vi "PH_Stepmotor_BaseClass.PC Relative Move.vi"(0 "i ref in":refnum<vi>, 1 "axis":i32=-1, 3 "Direction":T1, 4 "Multiple":i32=1, 5 "error in (no error)":errorcluster) -> (14 "i ref out":refnum<vi>, 19 "error out":errorcluster)   [LabVIEW 2014, in "PH_Stepmotor_BaseClass.lvlib"]
doc: "This VI calculates the target position and stores it own attributes."
uses:
  PH_Stepmotor_BaseClass.lvlib
  PH_Stepmotor_BaseClass.Axis Direction.ctl
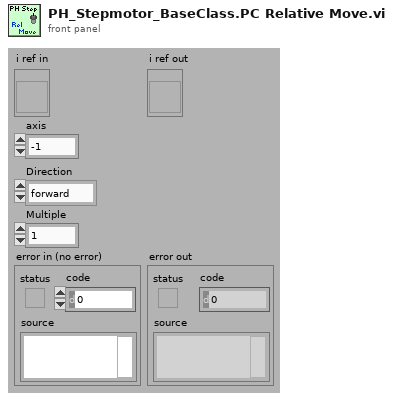
[diagram p1: front panel]
types:
  T1 = typedef "PH_Stepmotor_BaseClass.lvlib/PH_Stepmotor_BaseClass.Axis Direction.ctl" = enum16{"forward", "backward"}
  T2 = typedef "PH_Stepmotor_BaseClass.lvlib/PH_Stepmotor_BaseClass.Axis Attributes.ctl" = cluster{"Settings":T3, "Endswitch?":bool, "DIM Service IDs":T5, "Activity":T6, "Configured?":bool, "Position":cluster{"Current":i32, "Target":i32}, "Position to set":cluster{"New?":bool, "Wanted":i32}, "Stop?":bool, "Reset?":bool, "Move?":bool, "Nothing connected?":bool}
  T3 = typedef "PH_Stepmotor_BaseClass.lvlib/PH_Stepmotor_BaseClass.Axis Settings.ctl" = cluster{"Sign change":bool, "Width":dbl, "Calibration":dbl, "Unit":string, "Motor Type":T4, "Unit Width":string, "Unit CF":string}
  T4 = typedef "PH_Stepmotor_BaseClass.lvlib/PH_Stepmotor_BaseClass.Motor Type.ctl" = enum16{"Unspecific", "OWIS 49.120.2633", "OWIS 49.060.1033", "OWIS 43.040.2558", "Diamond Motion 2200 series", "OWIS 49.120.266B.MV6", "Calorimeter", "Linear Stage 1", "MICOS VT-80", "MICOS VT-80 S", "Standa Rotstage nt0.95A", "PUF RA 320.200", "PUF RA 800.200", "PUF RA 800.400", "PUF RA 400.50", "1324.nn.800.50", "1324.n9c.800.50", "1324.nn.320.200", "1324.nn.400.200", "1324.nn.800.200", "1324.nn.400.50", "1324.8c9c.800.50", "1324.8c9c.400.200"}
  T5 = typedef "PH_Stepmotor_BaseClass.lvlib/PH_Stepmotor_BaseClass.Axis DIM Service IDs.ctl" = cluster{"Settings":i32, "Information":i32}
  T6 = typedef "PH_Stepmotor_BaseClass.lvlib/PH_Stepmotor_BaseClass.Axis Activity.ctl" = enum16{"No Information", "stopped", "running", "Failure", "Alarm", "stopped at backward ES", "stopped at foreward ES"}
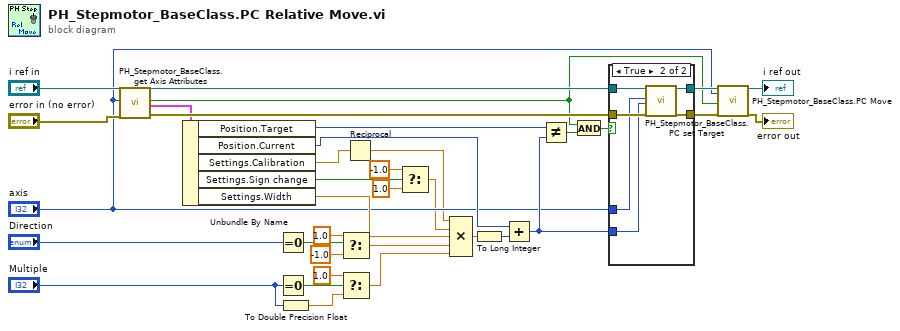
[diagram p0: block diagram]
diagram:
  n1 = call "PH_Stepmotor_BaseClass.get Axis Attributes.vi"("VI in"="i ref in", "Axis"="axis", "error in (no error)"="error in (no error)") -> ("VI out"=w32:refnum<vi>, "Axis found?"=w10:bool, "Axis Attributes"=w31:T2, "error out"=w34:errorcluster)  [unwired: 13 in]
  n2 = Unbundle By Name(w31) -> ("Position.Target"=w30:i32, "Position.Current"=w15:i32, "Settings.Calibration"=w8:dbl, "Settings.Sign change"=w19:bool, "Settings.Width"=w17:dbl)
  n3 = Equal To 0?(x="Direction") -> (x = 0?=w23:bool)
  n4 = Equal To 0?(x="Multiple") -> (x = 0?=w5:bool)
  n5 = To Double Precision Float(number="Multiple") -> (double precision float=w2:dbl)
  n6 = Select(t=1.0, s=w23, f=-1.0) -> (s? t:f=w22:dbl)
  n7 = Select(t=1.0, s=w5, f=w2) -> (s? t:f=w1:dbl)
  n8 = Reciprocal(x=w8) -> (1/x=w6:dbl)
  n9 = Select(t=-1.0, s=w19, f=1.0) -> (s? t:f=w7:dbl)
  n10 = Compound Arithmetic op=MULTIPLY(w6, w7, w17, w22, w1) -> (w21:dbl)
  n11 = To Long Integer(number=w21) -> (32bit integer=w16:i32)
  n12 = Add(x=w15, y=w16) -> (x+y=w20:i32)
  n13 = Not Equal?(x=w30, y=w20) -> (x != y?=w28:bool)
  n14 = And(x=w10, y=w28) -> (x .and. y?=w29:bool)
  n15 = case shown="True" w29 {
    tunnel: [w37 w38] -> w13
    tunnel: [w36 w39] -> w11
    tunnel: w34 -> [w36 w43]
    tunnel: w32 -> [w37 w42]
    tunnel: "axis" -> [_ w40]
    tunnel: w20 -> [_ w41]
    frame False {
    }
    frame True {
      n16 = call "PH_Stepmotor_BaseClass.PC set Target.vi"("VI in"=w42, "axis"=w40, "Targetposition to set"=w41, "error in (no error)"=w43) -> ("VI out"=w38:refnum<vi>, "error out"=w39:errorcluster)  [unwired: 14 in]
    }
  }
  n17 = call "PH_Stepmotor_BaseClass.PC Move.vi"("i ref in"=w13, "axis"="axis", "Move"=w10, "error in (no error)"=w11) -> ("i ref out"=→"i ref out":refnum<vi>, "error out"=→"error out":errorcluster)  [unwired: 14 in]
